vi "ROS_Topic_Close.vi"(0 "error in":errorcluster, 2 "topic":string, 3 "StopConsole":bool=TRUE) -> (1 "error out":errorcluster)   [LabVIEW 2013]
doc: "Closes a topic. If no topic is defined, it will close all tasks and close the console (unless specified otherwise)."
uses:
  _ROSDefinition.vi
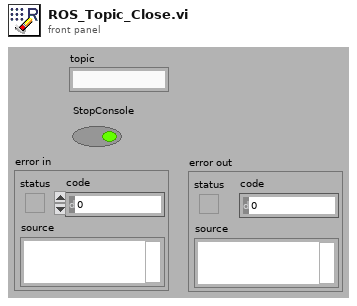
[diagram p1: front panel]
types:
  T1 = cluster{"server vi":string, "reference":refnum<vi>, "Description":string[], "Connected":bool}[]
  T2 = typedef "_ROSControl.ctl" = cluster{"topic port":u16, "Node":string, "topic":string, "type":string, "node port":u32, "error ":errorcluster, "Direction":T3, "APIs":string[]}
  T3 = typedef "_ROSDirection.ctl" = enum16{"Node", "Publisher", "Subscriber", "Service Client"}
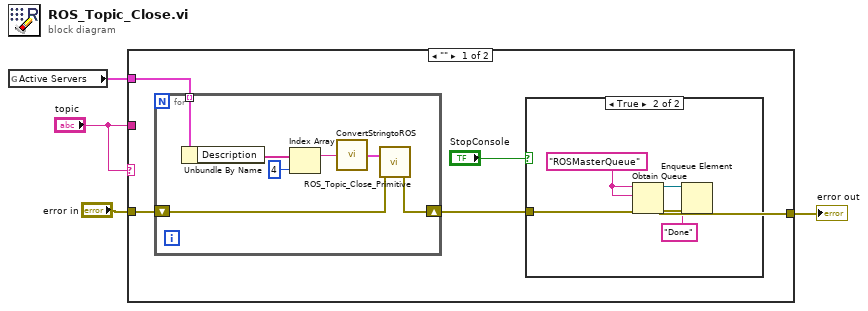
[diagram p0: block diagram]
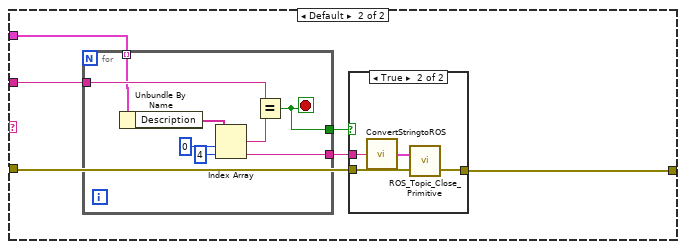
[diagram p3: hidden frame]
diagram:
  n1 = global read "_ROSDefinition.vi" "Active Servers"() -> (w1:T1)
  n2 = case shown="\"\"" "topic" {
    tunnel: "topic" -> [_ w25]
    tunnel: [w7 w23] -> w4
    tunnel: "error in" -> [w6 w22]
    tunnel: w1 -> [w5 w21]
    frame "" {
      n3 = for {
        shift-right: [w15] -> w7
        shift-left: w6 -> [w16]
        tunnel: w5 -> [w14] mode=indexing
        n4 = Unbundle By Name(w14) -> ("Description"=w20:string[])
        n5 = Index Array(array=w20, index=4) -> (element=w18:string)
        n6 = call "ConvertStringtoROS.vi"("string in"=w18) -> ("ROS"=w17:T2)
        n7 = call "ROS_Topic_Close_Primitive.vi"("error in"=w16, "ROS in"=w17) -> ("error out"=w15:errorcluster)  [unwired: 1 in]
      }
      n8 = case shown="True" "StopConsole" {
        tunnel: w7 -> [_ w10]
        frame False {
        }
        frame True {
          w12 = "ROSMasterQueue" ("name (unnamed)")
          n9 = Obtain Queue(name (unnamed)=w12, element data type=w12, error in (no error)=w10) -> (queue out=w13:refnum<queue>, error out=w9:errorcluster)  [unwired: 2 in, 1 out]
          n10 = Enqueue Element(queue=w13, element="Done", error in (no error)=w9) -> ()  [unwired: 1 in, 3 out]
        }
      }
    }
    frame Default {
      n11 = for {
        tunnel: [w36] -> w24
        tunnel: w25 -> [w34]
        tunnel: [w33] -> w26
        tunnel: w21 -> [w32] mode=indexing
        stop <- w33 stop-if-true
        n12 = Unbundle By Name(w32) -> ("Description"=w39:string[])
        n13 = Index Array(array=w39, index #1=0 ("index"), index #2=4 ("index")) -> (element #1=w35:string, element #2=w36:string)
        n14 = Equal?(x=w34, y=w35) -> (x = y?=w33:bool)
      }
      n15 = case shown="True" w26 {
        tunnel: w24 -> [_ w30]
        tunnel: [w27 w29] -> w23
        tunnel: w22 -> [w27 w28]
        frame False {
        }
        frame True {
          n16 = call "ConvertStringtoROS.vi"("string in"=w30) -> ("ROS"=w31:T2)
          n17 = call "ROS_Topic_Close_Primitive.vi"("error in"=w28, "ROS in"=w31) -> ("error out"=w29:errorcluster)  [unwired: 1 in]
        }
      }
    }
  }
  "error out" <- w4
